vi "Wojtyna_B_1.vi"   [LabVIEW 2020]
uses:
  <vilib>/Platform/TimedLoop/XDataNode/timing_clust.ctl
  <vilib>/Platform/TimedLoop/XDataNode/nitl_modes.ctl
  <vilib>/Platform/TimedLoop/XDataNode/wakeup.ctl
  <vilib>/platform/TimedLoop/XDataNode/XDataNode.xnode
  <vilib>/Platform/TimedLoop/XDataNode/XDNodeRunTimeDep.lvlib
types:
  T1 = typedef "XDNodeRunTimeDep.lvlib/timing_clust.ctl" = cluster{"Expected End [f-1]":u64, "Actual End [f-1]":u64, "Finished Late? [f-1]":bool, "Expected End [i-1]":u64, "Actual End [i-1]":u64, "Finished Late? [i-1]":bool, "Expected Start [i]":u64, "Actual Start [i]":u64, "Expected Start [f]":u64, "Actual Start [f]":u64, "Source Name":string, "Structure Name":string, "Period":i64, "Deadline":i64, "Offset":i64, "Start":i64, "Priority":i32, "Timeout":i32, "Mode":T2, "Wakeup Reason":T3, "Error":errorcluster, "Source Type":string, "Secondary Source Type":string, "Global End Time":u64, "Global Start Time":u64, "Frame Duration":u64, "Iteration Duration":u64, "Assigned CPU":i32, "I/O Scan Engine Mode":u32}
  T2 = typedef "XDNodeRunTimeDep.lvlib/nitl_modes.ctl" = enum32{"No Change", "Process missed periods, maintain original phase", "Discard missed periods, maintain original phase", "Process missed periods, ignore original phase", "Discard missed periods, ignore original phase"}
  T3 = typedef "XDNodeRunTimeDep.lvlib/wakeup.ctl" = enum32{"Normal", "Aborted", "Asynchronous wakeup", "Timing source error", "Timed loop error", "Timeout"}
  T4 = typedef "Rendezvous RefNum" = refnum<k1>
  T5 = typedef "Semaphore RefNum" = refnum<k1>
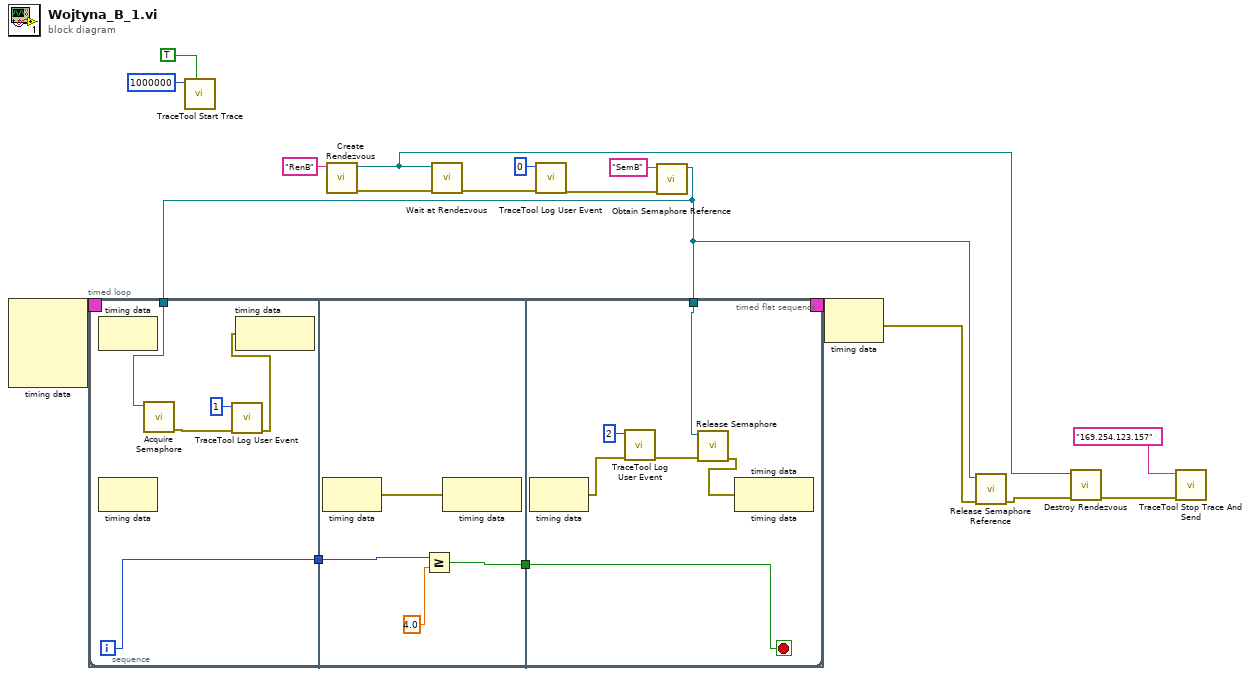
[diagram p0: block diagram]
diagram:
  n1 = node-c288() -> (w8:T1)  [unwired: 4 in]
  n2 = call <vilib>:"TraceTool Start Trace.vi"("Detailed Tracing? (F)"=TRUE, "Buffer Size (250000 bytes)"=1000000) -> ()  [unwired: 8 in, 2 out]
  n3 = call <vilib>:"Create Rendezvous.vi"("name (unnamed)"="RenB") -> ("error out"=w12:errorcluster, "rendezvous"=w4:T4)  [unwired: 4 in, 1 out]
  n4 = call <vilib>:"Wait at Rendezvous.vi"("error in (no error)"=w12, "rendezvous"=w4) -> ("error out"=w11:errorcluster)  [unwired: 3 in, 2 out]
  n5 = call <vilib>:"TraceTool Log User Event.vi"("error in (no error)"=w11, "Event ID (0-255)"=u32 0) -> ("error out"=w9:errorcluster)  [unwired: 9 in]
  n6 = call <vilib>:"Obtain Semaphore Reference.vi"("error in (no error)"=w9, "name (unnamed)"="SemB") -> ("semaphore"=w3:T5)  [unwired: 3 in, 2 out]
  n7 = timed-loop {
    timing: w8 -> [_]
    timing-out: [_] -> w7
    tunnel: w3 -> [w18]
    tunnel: w3 -> [w17]
    i -> [w24]
    stop <- w46 stop-if-true
    n8 = timed-sequence {
      timing: _ -> [_]
      timing-out: _ -> [_]
      tunnel: w18 -> [w22]
      tunnel: w17 -> [w19]
      n9 = timed-flat-sequence {
        tunnel: w22 -> [w27]
        tunnel: [w24] -> w21
        tunnel: w21 -> [w34]
        tunnel: [w33] -> w20
        tunnel: w20 -> [w46]
        tunnel: w19 -> [w42]
        frame #0 {
          n10 = node-c288() -> ()  [unwired: 1 in, 1 out]
          n11 = call <vilib>:"Acquire Semaphore.vi"("semaphore"=w27) -> ("error out"=w26:errorcluster)  [unwired: 4 in, 2 out]
          n12 = call <vilib>:"TraceTool Log User Event.vi"("error in (no error)"=w26, "Event ID (0-255)"=u32 1) -> ("error out"=w23:errorcluster)  [unwired: 9 in]
          n13 = node-c288(w23) -> ()  [unwired: 1 out]
        }
        frame #1 {
          n14 = node-c288() -> (w32:errorcluster)  [unwired: 1 in]
          n15 = Greater Or Equal?(x=w34, y=4.0) -> (x >= y?=w33:bool)
          n16 = node-c288(w32) -> ()  [unwired: 1 out]
        }
        frame #2 {
          n17 = node-c288() -> (w45:errorcluster)  [unwired: 1 in]
          n18 = call <vilib>:"TraceTool Log User Event.vi"("error in (no error)"=w45, "Event ID (0-255)"=u32 2) -> ("error out"=w43:errorcluster)  [unwired: 9 in]
          n19 = call <vilib>:"Release Semaphore.vi"("error in (no error)"=w43, "semaphore"=w42) -> ("error out"=w41:errorcluster)  [unwired: 4 in, 1 out]
          n20 = node-c288(w41) -> ()  [unwired: 1 out]
        }
      }
    }
    n21 = node-c288() -> ()  [unwired: 1 in, 1 out]
    n22 = node-c288() -> ()  [unwired: 1 in, 1 out]
  }
  n23 = node-c288(w7) -> (w6:errorcluster)
  n24 = call <vilib>:"Release Semaphore Reference.vi"("error in (no error)"=w6, "semaphore"=w3) -> ("error out"=w5:errorcluster)  [unwired: 8 in, 1 out]
  n25 = call <vilib>:"Destroy Rendezvous.vi"("error in (no error)"=w5, "rendezvous"=w4) -> ("error out"=w2:errorcluster)  [unwired: 4 in, 1 out]
  n26 = call <vilib>:"TraceTool Stop Trace And Send.vi"("error in (no error)"=w2, "Trace Host Network Address"="169.254.123.157") -> ()  [unwired: 9 in, 1 out]
